vi "Config-BaudRate.vi"(8 "error in (no error)":errorcluster, 10 "Def-PreConfig-BaudRate":T1={"Channel Num"=0, "BaudRate"=125000} {"BaudRate" items=["1 MBaud"=1000000, "800 KBaud"=800000, "500 KBaud"=500000, "400 KBaud"=400000, "250 KBaud"=250000, "200 KBaud"=200000, "160 KBaud"=160000, "125 KBaud"=125000, "100 KBaud"=100000, "83.3 KBaud"=83333, "80 KBaud"=80000, "62.5 KBaud"=62500, "50 KBaud"=50000, "40 KBaud"=40000, "33.3 KBaud"=33333, "<Custom>"=0]}, 11 "CAN-NI in":refnum<class "CAN-NI.lvclass">) -> (0 "error out":errorcluster, 3 "CAN-NI out":refnum<class "CAN-NI.lvclass">)   [LabVIEW 2019, in "CAN-NI.lvlib" / "CAN-NI.lvclass"]
uses:
  CAN-NI.lvclass
  CAN-Interface/TypeDef/Def-Config-BaudRate.ctl
  CAN-Interface/TypeDef/Def-BaudRate.ctl
  <resource>/objmgr/xnet.rc
  CAN-Interface/Class-Interface.lvclass
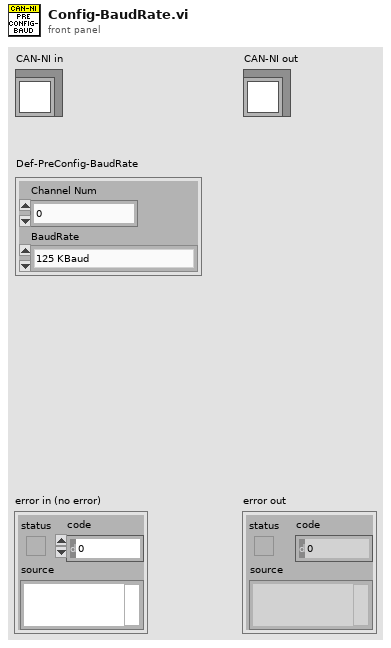
[diagram p1: front panel]
types:
  T1 = typedef "CAN-Interface.lvlib/Class-Interface.lvclass/Def-Config-BaudRate.ctl" = cluster{"Channel Num":u32, "BaudRate":T2}
  T2 = typedef "CAN-Interface.lvlib/Class-Interface.lvclass/Def-BaudRate.ctl" = u32
  T3 = typedef "CAN-NI.lvlib/CAN-NI.lvclass/ChannelProperty.ctl" = cluster{"CAN-cluster":refnum<k21>, "CAN-Frames":refnum<k21>[], "Termination":T4, "Transmit Mode":T5, "Frame Out Session":refnum<k21>, "Frame In Session":refnum<k21>, "Protocol":T6}
  T4 = typedef "CAN-Interface.lvlib/Class-Interface.lvclass/Def-Termination.ctl" = enum8{"on", "off"}
  T5 = typedef "CAN-Interface.lvlib/Class-Interface.lvclass/Def-Transmit Mode.ctl" = enum16{"Queued", "Stream"}
  T6 = typedef "CAN-Interface.lvlib/Class-Interface.lvclass/Def-Protocol.ctl" = enum16{"CAN", "CAN FD"}
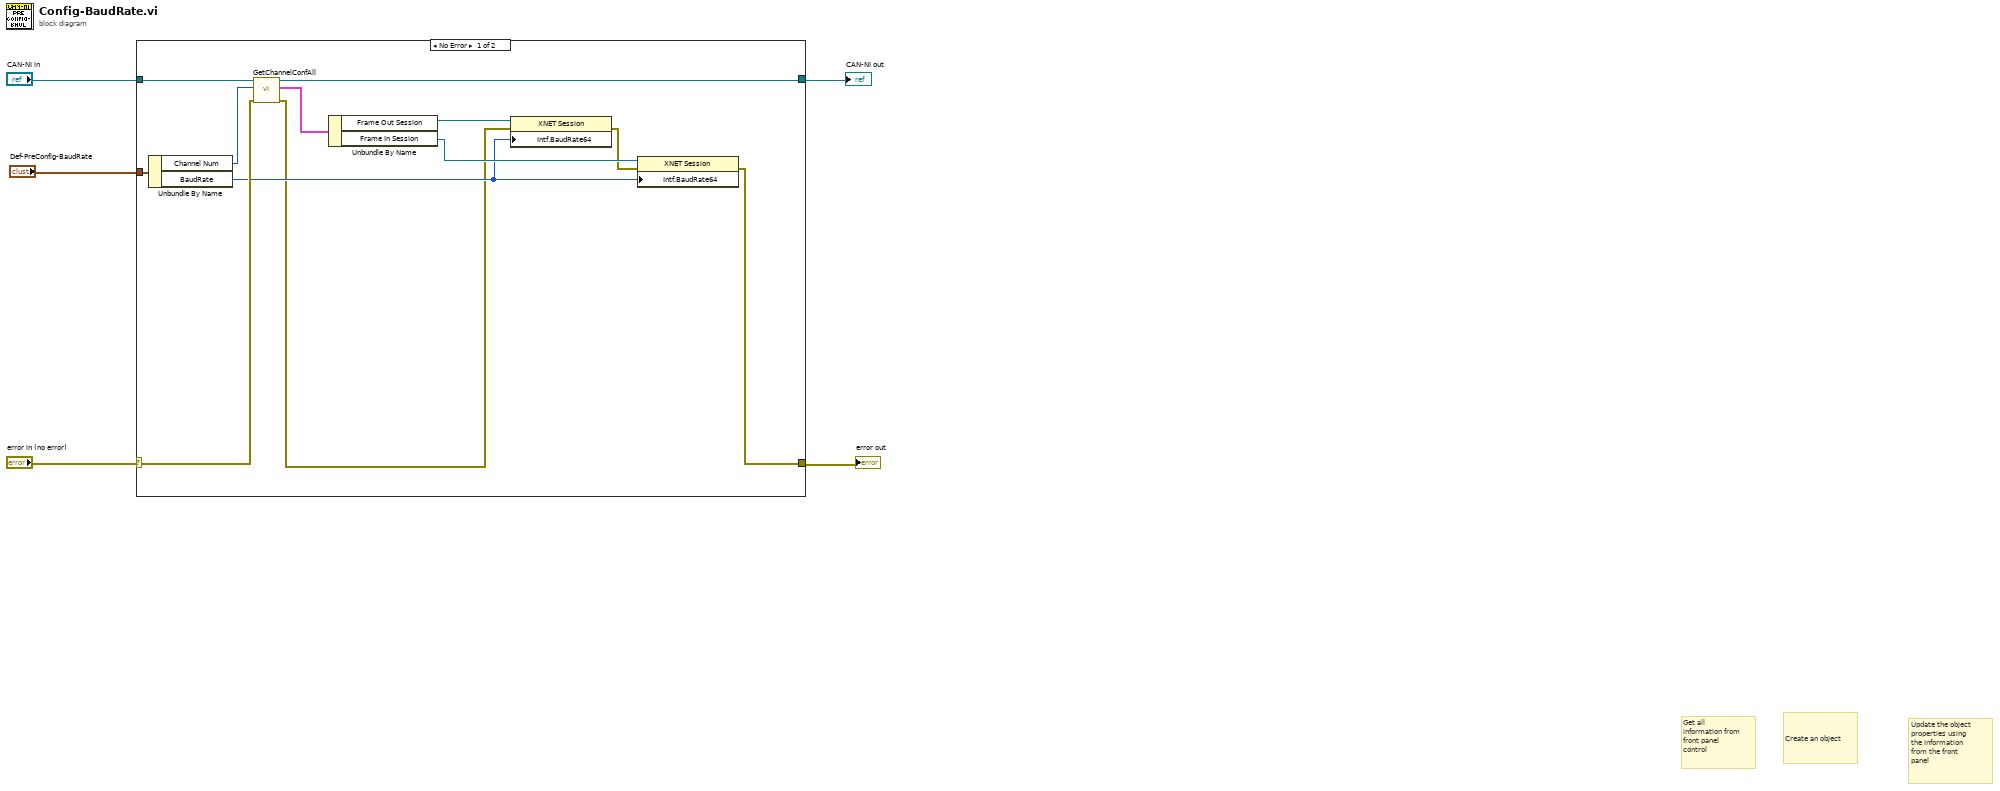
[diagram p0: block diagram]
diagram:
  # "Update the object properties using the information from the front panel"
  # "Create an object"
  # "Get all information from front panel control"
  n1 = case shown="No Error" "error in (no error)" {
    selector: "error in (no error)" -> [w13 w18]
    tunnel: [w6 w18] -> w4
    tunnel: "CAN-NI in" -> [w15 w19]
    tunnel: [w14 w19] -> w2
    tunnel: "Def-PreConfig-BaudRate" -> [w17 _]
    frame No Error {
      n2 = Unbundle By Name(w17) -> ("Channel Num"=w16:u32, "BaudRate"=w9:T2)
      n3 = call "GetChannelConfAll.vi"("error in"=w13, "Channel Num"=w16, "CAN-NI"=w15) -> ("error out"=w8:errorcluster, "ChannelProperty"=w12:T3, "CAN-NI"=w14:refnum<class "CAN-NI.lvclass">)  [unwired: 6 in]
      n4 = Unbundle By Name(w12) -> ("Frame Out Session"=w11:refnum<k21>, "Frame In Session"=w10:refnum<k21>)
      n5 = property class="XNET Session"(reference=w11, error in=w8, "Intf.BaudRate64"=w9) -> (error out=w7:errorcluster)  [unwired: 1 out]
      n6 = property class="XNET Session"(reference=w10, error in=w7, "Intf.BaudRate64"=w9) -> (error out=w6:errorcluster)  [unwired: 1 out]
    }
    frame Error {
    }
  }
  "error out" <- w4
  "CAN-NI out" <- w2
